vi "CP和UA计算.vi"(11 "数组":string[][](array[string])) -> (2 "cp":dbl, 3 "UA":dbl)   [LabVIEW 2023]
uses:
  <vilib>/Analysis/NI_AALPro.lvlib
  <vilib>/Analysis/NI_AAL_SigProc.lvlib
  <vilib>/Analysis/NI_AALBase.lvlib
  <vilib>/Analysis/baseanly.llb/Mean (DBL).vi
  <vilib>/Analysis/8numeric.llb/1D Numeric Integration.vi
panel:
  in  "反应液质量":dbl
  in  "材料常数":dbl
  out "上升3℃的部分":dbl[][](array[numeric])
  out "提出的300个点的数组":dbl[][](array[numeric])
  out "去除基线后的波形":dbl[][](array[numeric])
  out "原始波形":dbl[][](array[numeric])
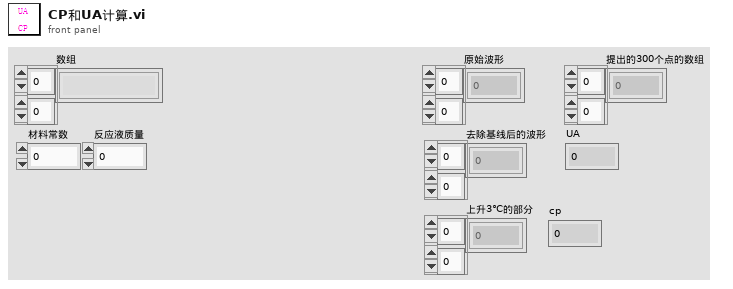
[diagram p1: front panel]
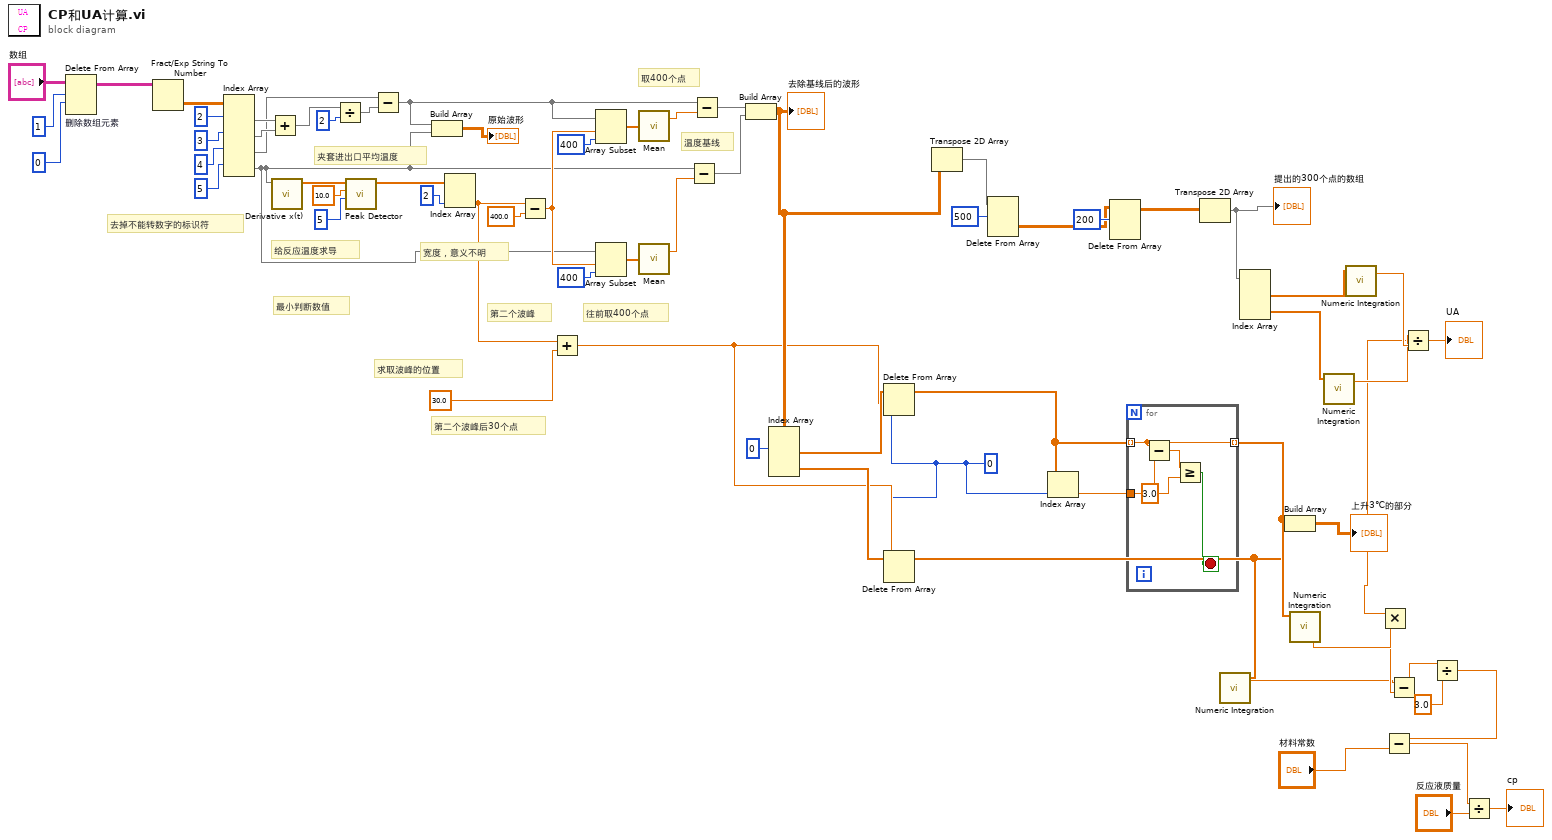
[diagram p0: block diagram]
diagram:
  w17 = 0 ("索引 (行)")
  # "第二个波峰后30个点"
  # "往前取400个点"
  # "温度基线"
  # "取400个点"
  # "宽度，意义不明"
  # "最小判断数值"
  # "第二个波峰"
  # "求取波峰的位置"
  # "给反应温度求导"
  # "夹套进出口平均温度"
  # "去掉不能转数字的标识符"
  n1 = Delete From Array "删除数组元素"(array="数组", length=1 ("禁用的索引 (列)"), index (row)=0 ("禁用的索引 (列)")) -> (array with subset deleted=w65:string[][])  [unwired: 1 in, 1 out]
  n2 = Fract/Exp String To Number(string=w65) -> (number=w63:dbl[][])  [unwired: 3 in, 1 out]
  n3 = Index Array(array=w63, index (row) #1=2 ("索引 (行)"), index (row) #2=3 ("索引 (行)"), index (row) #3=4 ("索引 (行)"), index (row) #4=5 ("索引 (行)")) -> (element #1=w58:dbl[], element #2=w57:dbl[], element #3=w50:dbl[], element #4=w37:dbl[])  [unwired: 4 in]
  n4 = Add(x=w58, y=w57) -> (x+y=w56:dbl[])
  n5 = call <vilib>:"Derivative x(t).vi"("X"=w37) -> ("dX/dt"=w54:dbl[])  [unwired: 9 in, 1 out]
  n6 = Divide(x=w56, y=2) -> (x/y=w49:dbl[])
  n7 = call <vilib>:"Peak Detector.vi"("width"=5, "threshold"=10.0, "X"=w54) -> ("Locations"=w35:dbl[])  [unwired: 4 in, 4 out]
  n8 = Subtract(x=w50, y=w49) -> (x-y=w43:dbl[])
  n9 = Build Array(w43, w37) -> (→"原始波形":dbl[][])
  n10 = Index Array(array=w35, index #2=2 ("索引")) -> (element #2=w19:dbl)  [unwired: 1 in, 1 out]
  n11 = Subtract(x=w19, y=400.0) -> (x-y=w41:dbl)
  n12 = Add(x=w19, y=30.0) -> (x+y=w18:dbl)
  n13 = Array Subset(array=w43, index=w41, length=400 ("长度")) -> (w46:dbl[])
  n14 = Array Subset(array=w37, index=w41, length=400 ("长度")) -> (w39:dbl[])
  n15 = call-poly <vilib>:"Mean.vi"("X"=w46) -> ("mean"=w44:dbl)  [unwired: 1 out]
  n16 = call-poly <vilib>:"Mean.vi"("X"=w39) -> ("mean"=w38:dbl)  [unwired: 1 out]
  n17 = Subtract(x=w37, y=w38) -> (x-y=w36:dbl[])
  n18 = Subtract(x=w43, y=w44) -> (x-y=w42:dbl[])
  n19 = Build Array(w42, w36) -> (w23:dbl[][])
  "去除基线后的波形" <- w23
  n20 = Index Array(array=w23, index (row) #1=0 ("索引 (行)")) -> (element #1=w21:dbl[], element #2=w20:dbl[])  [unwired: 3 in]
  n21 = Delete From Array(array=w21, length=w18, index=w17) -> (array with subset deleted=w16:dbl[])  [unwired: 1 out]
  n22 = Delete From Array(array=w20, length=w18, index=w17) -> (array with subset deleted=w12:dbl[])  [unwired: 1 out]
  n23 = Transpose 2D Array(2D array=w23) -> (transposed array=w33:dbl[][])
  n24 = Delete From Array(array=w33, length=500 ("长度")) -> (deleted portion=w30:dbl[][])  [unwired: 2 in, 1 out]
  n25 = Index Array(array=w16, index=w17) -> (element=w15:dbl)
  n26 = Delete From Array(array=w30, length=200 ("长度")) -> (array with subset deleted=w29:dbl[][])  [unwired: 2 in, 1 out]
  n27 = for {
    tunnel: w16 -> [w68] mode=indexing
    tunnel: w15 -> [w70]
    tunnel: [w68] -> w13 mode=indexing
    stop <- w69 stop-if-true
    n28 = Subtract(x=w68, y=w70) -> (x-y=w71:dbl)
    n29 = Greater Or Equal?(x=w71, y=3.0) -> (x >= y?=w69:bool)
  }
  n30 = Transpose 2D Array(2D array=w29) -> (transposed array=w28:dbl[][])
  "提出的300个点的数组" <- w28
  n31 = call-poly <vilib>:"Numeric Integration.vi"("Input Array"=w12) -> ("result"=w8:dbl)  [unwired: 2 in, 1 out]
  n32 = Index Array(array=w28) -> (element #1=w27:dbl[], element #2=w26:dbl[])  [unwired: 4 in]
  n33 = Build Array(w13, w12) -> (→"上升3℃的部分":dbl[][])
  n34 = call-poly <vilib>:"Numeric Integration.vi"("Input Array"=w13) -> ("result"=w11:dbl)  [unwired: 2 in, 1 out]
  n35 = call-poly <vilib>:"Numeric Integration.vi"("Input Array"=w26) -> ("result"=w24:dbl)  [unwired: 2 in, 1 out]
  n36 = call-poly <vilib>:"Numeric Integration.vi"("Input Array"=w27) -> ("result"=w25:dbl)  [unwired: 2 in, 1 out]
  n37 = Divide(x=w24, y=w25) -> (x/y=w10:dbl)
  "UA" <- w10
  n38 = Multiply(x=w10, y=w11) -> (x*y=w9:dbl)
  n39 = Subtract(x=w8, y=w9) -> (x-y=w7:dbl)
  n40 = Divide(x=w7, y=3.0) -> (x/y=w5:dbl)
  n41 = Subtract(x=w5, y="材料常数") -> (x-y=w3:dbl)
  n42 = Divide(x=w3, y="反应液质量") -> (x/y=→"cp":dbl)
